vi "Do.vi"(8 "error in (no error)":errorcluster, 10 "Actor in":refnum<class "Actor.lvclass">, 11 "AsynchReturnMsg":refnum<class "CS++AsynchReturnMsg.lvclass">) -> (0 "error out":errorcluster, 2 "Actor out":refnum<class "Actor.lvclass">)   [LabVIEW 2016, in "CS++AsynchReturnMsg.lvlib" / "CS++AsynchReturnMsg.lvclass"]
doc: "(<B>Filename</B>: Actor Framework.lvlib:Message.lvclass:Do.vi)\n\nDefines what a message does when it is received by an actor. Generally, a message instructs an actor to invoke one of its methods. By default, this method does nothing. A child class must override it to define behavior. Create a child class by using the Actor Framework Message Maker dialog box."
uses:
  CS++AsynchReturnMsg.lvclass
  <vilib>/ActorFramework/Actor/Actor.lvclass
  CS++AsynchReturnMsg.lvclass/CS++AsynchReturnMsg.ctl
  CS++AcknowledgeMsg/CS++AcknowledgeMsg.lvclass/CS++AcknowledgeMsg.ctl
  <vilib>/ActorFramework/Message Enqueuer/Message Enqueuer.lvclass/Message Enqueuer.ctl
  Libraries/Base/Severity.ctl
  <vilib>/ActorFramework/Message Enqueuer/Enqueue.vi
  CS++AcknowledgeMsg/CS++AcknowledgeMsg.lvclass
  C:/Program Files (x86)/National Instruments/LabVIEW 2016/vi.lib/ActorFramework/Message/Message.lvclass
  <vilib>/ActorFramework/Message Priority Queue/Priority Enqueue.vi
  <vilib>/ActorFramework/Message Enqueuer/Message Enqueuer.lvclass
  Libraries/Utilities/CS++Utilities.lvlib
  Libraries/Base/CS++Base.lvlib
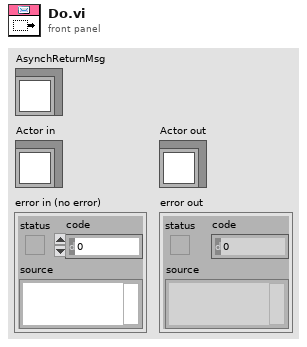
[diagram p1: front panel]
types:
  T1 = typedef "CS++Base.lvlib/Severity.ctl" = enum16{"emergency", "alert", "critical", "error", "warning", "notice", "info", "debug"}
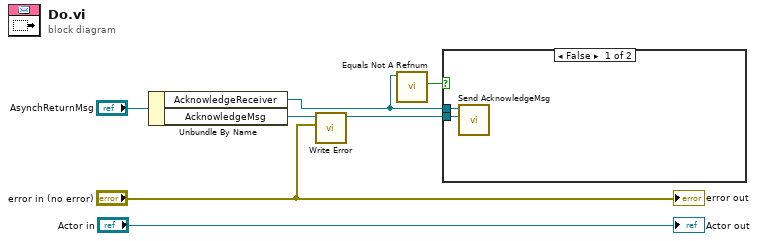
[diagram p0: block diagram]
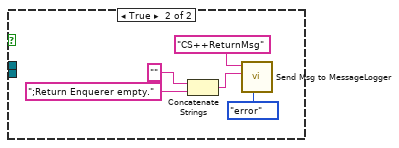
[diagram p2: hidden frame]
diagram:
  n1 = Unbundle By Name("AsynchReturnMsg") -> ("AcknowledgeReceiver"=w2:refnum<class "Message Enqueuer.lvclass">, "AcknowledgeMsg"=w5:refnum<class "CS++AcknowledgeMsg.lvclass">)
  n2 = call "Write Error.vi"("Error"="error in (no error)", "AcknowledgeMsg in"=w5) -> ("AcknowledgeMsg out"=w3:refnum<class "CS++AcknowledgeMsg.lvclass">)  [unwired: 8 in, 1 out]
  n3 = call <vilib>:"Equals Not A Refnum.vi"("Message Enqueuer"=w2) -> ("Not a refnum?"=w1:bool)  [unwired: 10 in]
  n4 = case shown="False" w1 {
    tunnel: w3 -> [w9 _]
    tunnel: w2 -> [w8 _]
    frame False {
      n5 = call "Send AcknowledgeMsg.vi"("Acknowledge Msg"=w9, "Message Enqueuer"=w8) -> ()  [unwired: 8 in, 2 out]
    }
    frame True {
      n6 = Concatenate Strings("" ("string"), ";Return Enquerer empty." ("Message Tag")) -> (w12:string)
      n7 = call "Send Msg to MessageLogger.vi"("Severity Code (info)"=Severity."error", "Message Content"=w12, "Message Tag"="CS++ReturnMsg") -> ()  [unwired: 8 in, 1 out]
    }
  }
  "error out" <- "error in (no error)"
  "Actor out" <- "Actor in"
